vi "8 swich.vi"() -> ()   [LabVIEW 2017]
panel:
  out "Gauge":dbl(knob) scale=0.0..256.0
  out "Slide":u8(slide) scale=0.0..256.0
  out "Numeric":i16
  in  "Boolean 11":bool
  in  "Boolean 10":bool
  in  "Boolean 9":bool
  in  "Boolean 8":bool
  in  "Boolean 7":bool
  in  "Boolean 6":bool
  in  "Boolean 5":bool
  in  "Boolean 4":bool
  in  "stop":bool
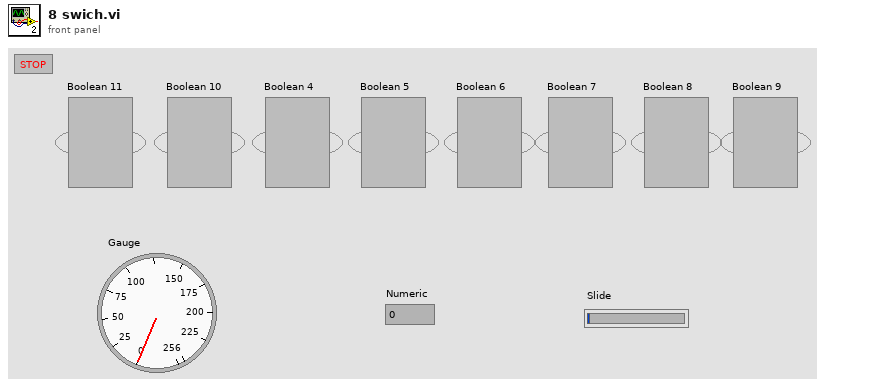
[diagram p1: front panel]
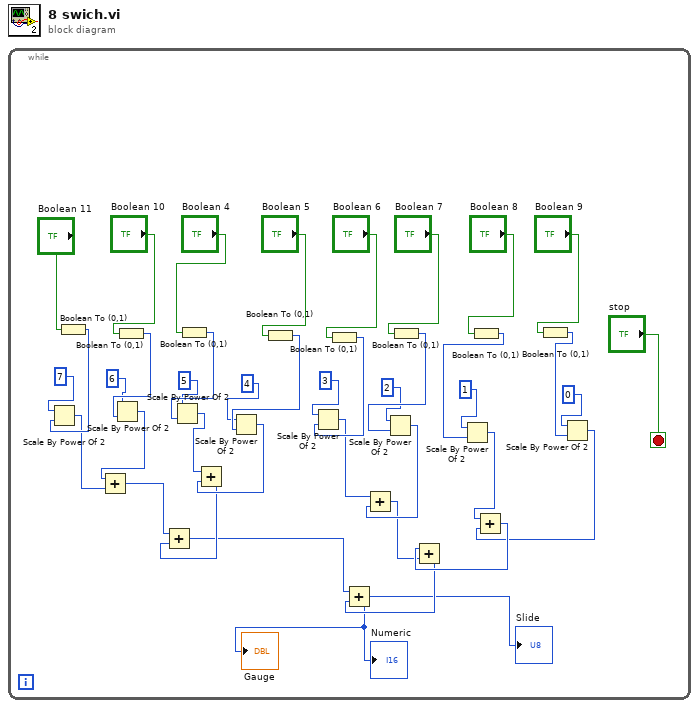
[diagram p0: block diagram]
diagram:
  n1 = while {
    stop <- "stop" stop-if-true
    n2 = Boolean To (0,1)(Boolean="Boolean 11") -> (0, 1=w17:i16)
    n3 = Scale By Power Of 2(n=7, x=w17) -> (x*2^n=w16:i16)
    n4 = Boolean To (0,1)(Boolean="Boolean 10") -> (0, 1=w38:i16)
    n5 = Scale By Power Of 2(n=6, x=w38) -> (x*2^n=w15:i16)
    n6 = Add(x=w15, y=w16) -> (x+y=w12:i16)
    n7 = Boolean To (0,1)(Boolean="Boolean 4") -> (0, 1=w35:i16)
    n8 = Scale By Power Of 2(n=5, x=w35) -> (x*2^n=w14:i16)
    n9 = Boolean To (0,1)(Boolean="Boolean 5") -> (0, 1=w32:i16)
    n10 = Scale By Power Of 2(n=4, x=w32) -> (x*2^n=w13:i16)
    n11 = Add(x=w14, y=w13) -> (x+y=w4:i16)
    n12 = Add(x=w12, y=w4) -> (x+y=w3:i16)
    n13 = Boolean To (0,1)(Boolean="Boolean 6") -> (0, 1=w28:i16)
    n14 = Scale By Power Of 2(n=3, x=w28) -> (x*2^n=w11:i16)
    n15 = Boolean To (0,1)(Boolean="Boolean 7") -> (0, 1=w26:i16)
    n16 = Scale By Power Of 2(n=2, x=w26) -> (x*2^n=w10:i16)
    n17 = Add(x=w11, y=w10) -> (x+y=w8:i16)
    n18 = Boolean To (0,1)(Boolean="Boolean 8") -> (0, 1=w23:i16)
    n19 = Scale By Power Of 2(n=1, x=w23) -> (x*2^n=w6:i16)
    n20 = Boolean To (0,1)(Boolean="Boolean 9") -> (0, 1=w19:i16)
    n21 = Scale By Power Of 2(n=0, x=w19) -> (x*2^n=w5:i16)
    n22 = Add(x=w6, y=w5) -> (x+y=w9:i16)
    n23 = Add(x=w9, y=w8) -> (x+y=w7:i16)
    n24 = Add(x=w3, y=w7) -> (x+y=→"Slide" →"Gauge" →"Numeric":i16)
  }
